vi "Analyse Data_SubVI.vi"(8 "error in (no error)":errorcluster, 11 "Data in":dbl[](array[numeric])) -> (0 "error out":errorcluster)   [LabVIEW 2020]
uses:
  <vilib>/Analysis/baseanly.llb/Mean (DBL).vi
  <vilib>/Analysis/NI_AALBase.lvlib
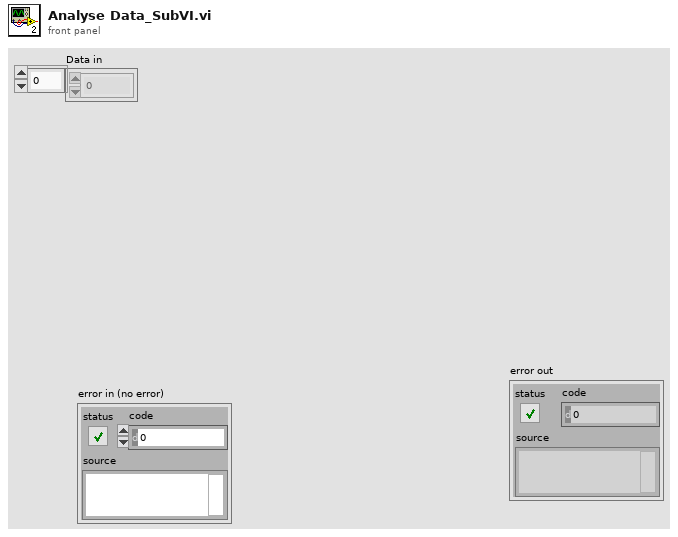
[diagram p1: front panel]
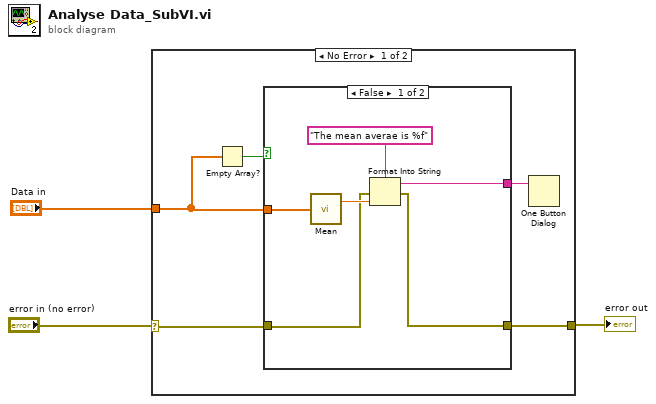
[diagram p0: block diagram]
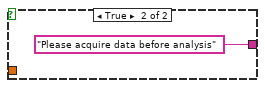
[diagram p2: hidden frame]
diagram:
  n1 = case shown="No Error" "error in (no error)" {
    selector: "error in (no error)" -> [w5 w16]
    tunnel: [w4 w16] -> w2
    tunnel: "Data in" -> [w6 _]
    frame No Error {
      n2 = Empty Array?(array=w6) -> (empty?=w8:bool)
      n3 = case shown="False" w8 {
        tunnel: [w13 "Please acquire data before analysis"] -> w7
        tunnel: w6 -> [w14 _]
        tunnel: w5 -> [w10 _]
        tunnel: [w9 _] -> w4
        frame False {
          n4 = call-poly <vilib>:"Mean.vi"("X"=w14) -> ("mean"=w12:dbl)  [unwired: 1 out]
          n5 = Format Into String(format string="The mean averae is %f", error in=w10, w12) -> (resulting string=w13:string, error out=w9:errorcluster)  [unwired: 1 in]
        }
        frame True {
        }
      }
      n6 = One Button Dialog(message=w7) -> ()  [unwired: 1 in, 1 out]
    }
    frame Error {
    }
  }
  "error out" <- w2
